vi "Resolve-client-from-channel.vi"(8 "error in (no error)":errorcluster, 10 "Client channel":refnum<queue>) -> (0 "error out":errorcluster, 1 "Client ID":i32, 2 "Client type":T1)   [LabVIEW 2013, in "CameraVision.lvlib" / "CV-Client.lvclass"]
uses:
  CV-Client.lvclass
  SA-SLMAPI/Sources/Message.lvclass
  Supported-modules.ctl
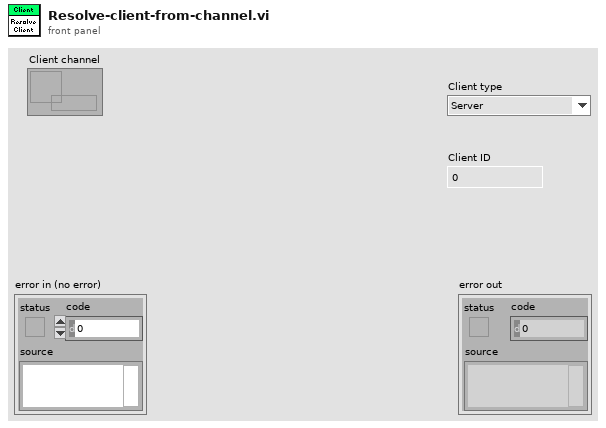
[diagram p1: front panel]
types:
  T1 = typedef "CameraVision.lvlib/CV-Client.lvclass/Supported-modules.ctl" = enum16{"Server", "All", "SLMControl", "PowderDeposition", "StrategyParser", "CameraVision", "MaterialCharacterization", "StatusMonitor", "SLMSimulation", "LaserCharacterization"}
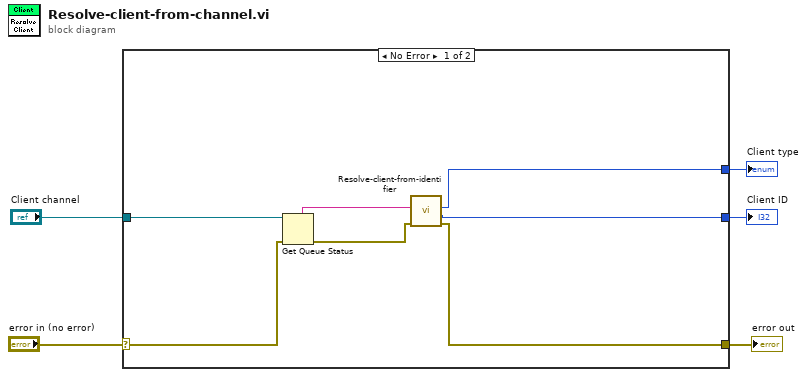
[diagram p0: block diagram]
diagram:
  n1 = case shown="No Error" "error in (no error)" {
    selector: "error in (no error)" -> [w11 w13]
    tunnel: [w8 w13] -> w4
    tunnel: "Client channel" -> [w12 _]
    tunnel: [w7 _] -> w2
    tunnel: [w6 _] -> w1
    frame No Error {
      n2 = Get Queue Status(queue=w12, error in (no error)=w11) -> (queue name=w10:string, error out=w9:errorcluster)  [unwired: 1 in, 6 out]
      n3 = call "Resolve-client-from-identifier.vi"("error in (no error)"=w9, "Client identifier"=w10) -> ("error out"=w8:errorcluster, "Client ID"=w6:i32, "Client type"=w7:T1)  [unwired: 7 in]
    }
    frame Error {
    }
  }
  "error out" <- w4
  "Client type" <- w2
  "Client ID" <- w1
